vi "Exposure Mode to String.vi"(1 "Exp Mode":T1) -> (0 "String":string)   [LabVIEW 2020, in "Camera.lvclass"]
uses:
  Camera.lvclass
  Camera.lvclass/Camera.ctl
  Exposure Mode.ctl
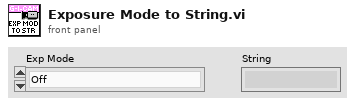
[diagram p1: front panel]
types:
  T1 = typedef "Camera.lvclass/Exposure Mode.ctl" = enum8{"Off", "Timed", "Trigger Width", "Trigger Controller"}
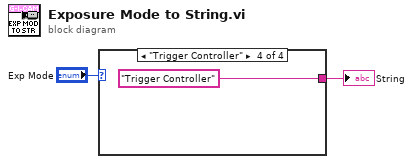
[diagram p0: block diagram]
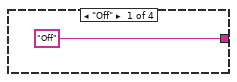
[diagram p2: hidden frame]
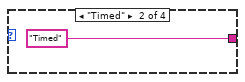
[diagram p3: hidden frame]
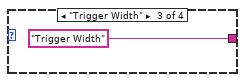
[diagram p4: hidden frame]
diagram:
  n1 = case shown="\"Trigger Controller\"" "Exp Mode" {
    tunnel: ["Off" "Timed" "Trigger Width" "Trigger Controller"] -> w1
    frame "Off" {
    }
    frame "Timed" {
    }
    frame "Trigger Width" {
    }
    frame "Trigger Controller" {
    }
  }
  "String" <- w1
